vi "Read-all-gui-params.vi"(8 "error in (no error)":errorcluster, 11 "Storage params. ref. in":refnum<data-value>) -> (0 "error out":errorcluster, 2 "Storage params.":T1={"Base file name"="Test", "Storage directory"=path "C:/CameraVision/Results", "Save what?"={"Original"=FALSE, "Corrected"=FALSE, "Binary"=FALSE, "Temperature"=FALSE, "Characteristics"=FALSE, "Mapping"=FALSE, "TemperatureValues"=FALSE}, "Image file type"=enum."BMP", "Comments"="", "Storage mode"=enum."1 file for all layers ", "Start iteration/layer"=0}, 3 "Storage params. ref.":refnum<data-value>)   [LabVIEW 2013, in "CameraVision.lvlib" / "CV-Storage.lvclass"]
uses:
  CV-Storage.lvclass
  Storage-parameters-gui.ctl
  Storage-types.ctl
  CV-Storage.lvclass/CV-Storage.ctl
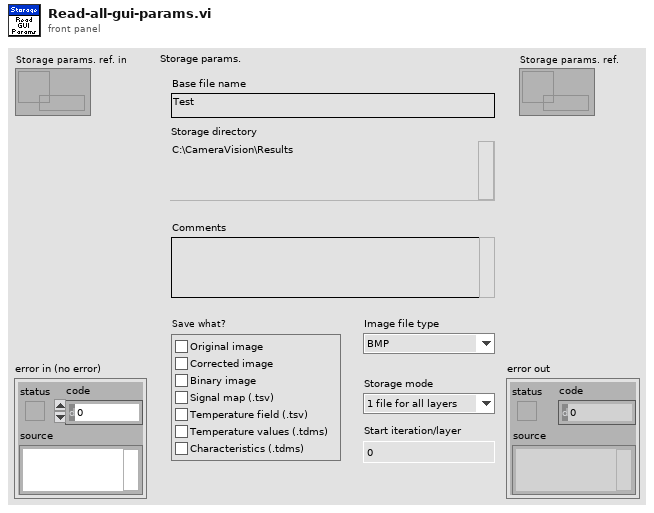
[diagram p1: front panel]
types:
  T1 = typedef "CameraVision.lvlib/CV-Storage.lvclass/Storage-parameters-gui.ctl" = cluster{"Base file name":string, "Storage directory":path, "Save what?":T2, "Image file type":enum16{"JPG", "BMP", "PNG"}, "Comments":string, "Storage mode":enum16{"1 file per layer", "1 file for all layers "}, "Start iteration/layer":u16}
  T2 = typedef "CameraVision.lvlib/CV-Storage.lvclass/Storage-types.ctl" = cluster{"Original":bool, "Corrected":bool, "Binary":bool, "Temperature":bool, "Characteristics":bool, "Mapping":bool, "TemperatureValues":bool}
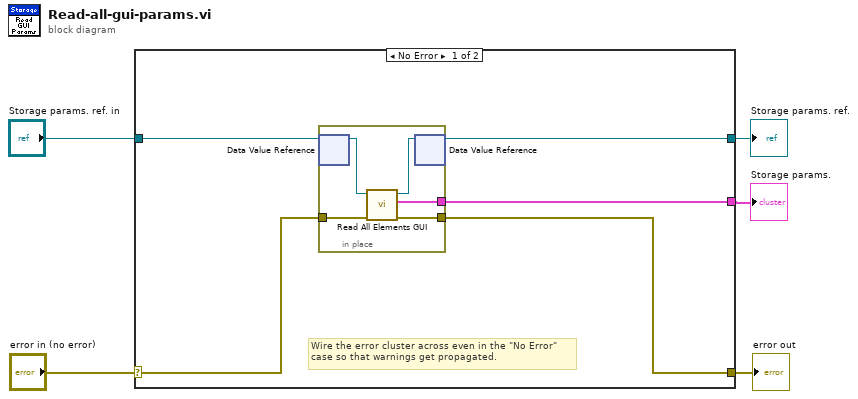
[diagram p0: block diagram]
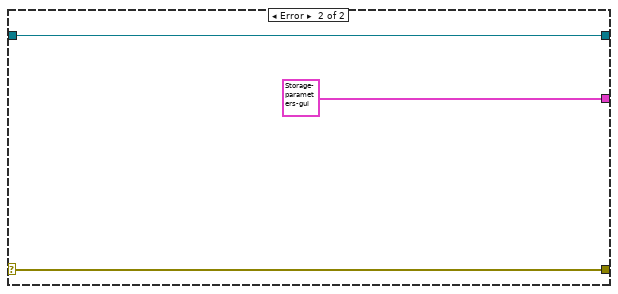
[diagram p2: hidden frame]
diagram:
  n1 = case shown="No Error" "error in (no error)" {
    selector: "error in (no error)" -> [w8 w18]
    tunnel: [w10 w18] -> w4
    tunnel: "Storage params. ref. in" -> [w7 w16]
    tunnel: [w9 T1 {"Base file name"="Test", "Storage directory"=path "C:/CameraVision/Results", "Save what?"={"Original"=FALSE, "Corrected"=FALSE, "Binary"=FALSE, "Temperature"=FALSE, "Characteristics"=FALSE, "Mapping"=FALSE, "TemperatureValues"=FALSE}, "Image file type"=enum."BMP", "Comments"="", "Storage mode"=enum."1 file per layer", "Start iteration/layer"=0} ("Storage params.")] -> w2
    tunnel: [w6 w16] -> w1
    frame No Error {
      # "Wire the error cluster across even in the \"No Error\"\ncase so that warnings get propagated."
      n2 = in-place {
        in-place-border: [w15] -> w10
        in-place-border: [w14] -> w9
        in-place-border: w8 -> [w13]
        n3 = in-place-dvr #1(w7) -> (w11:refnum<class "CV-Storage.lvclass">)  [unwired: 1 out]
        n4 = call "Read All Elements GUI.vi"("error in (no error)"=w13, "Storage params in"=w11) -> ("error out"=w15:errorcluster, "Storage params."=w14:T1, "Storage params out"=w12:refnum<class "CV-Storage.lvclass">)  [unwired: 7 in]
        n5 = in-place-dvr #1(w12) -> (w6:refnum<data-value>)  [unwired: 1 out]
      }
    }
    frame Error {
    }
  }
  "error out" <- w4
  "Storage params. ref." <- w1
  "Storage params." <- w2
